vi "Dictionary Example.vi"() -> ()   [LabVIEW 2020]
uses:
  <userlib>/_OpenG.lib/dictionary/dictionary.llb/Dictionary Update (by scalar value)__ogtk.vi
  <userlib>/_OpenG.lib/string/string.llb/Trim Whitespace (String)__ogtk.vi
panel:
  in  "Copyright":bool
  in  "Help":bool
  in  "Cancel":bool
  in  "Delete Selected User":bool
  in  "Add":bool
  in  "New Username":string
  in  "Add New User":bool
  in  "Revert":bool
  in  "Exit":bool
  in  "Apply":bool
  in  "User Information":cluster{"Country":string, "Age":i32}
  out "error out":errorcluster
  in  "Selected User":u16(ring) items=["<Select Username>", "Tom", "Harish", "Sam", "Ghulam", "Henry", "Jon"]
  in  "error in (no error)":errorcluster
  # "Instructions to use the example:\n\n1. <Display User Information>\n     Select the User from \"Select User\" dropdown listbox\n     The information of that user will be displayed in \"User Information\" section\n\n2. <Modify User Information>\n     Select the User from \"Select User\" dropdown listbox\n     Modify the User Information\n     Click \"Apply Changes\" button to save\n\n3. <Revert User Information Changes>\n     Click \"Revert\" button to cancel the modifications\n\n3. <Add New User>\n    Click \"Add new user\" button\n    Enter the new user name in \"New Username\" button \n    Press \"+\" button to add       \n    the username to the dictionary\n\n4. <Delete Existing Username>\n     Select the username in \"Selected User\" listbox\n     Click \"Delete Selected User\" button\n     Select \"Yes\" in the confirmation dialog window\n\n5. <Exit>\n     Click \"Exit\" button to exit the application\n\n6. <Help>\n     Click \"Help\"button to see this help text in a dialog box."
  # "<Dictionary Example.vi> - <Demonstrates use of OpenG Dictionary functions>\n\nCopyright (C) 2005 Ashish Uttarwar <ashish.uttarwar@jameskring.com>\nCopyright (C) 2010 Jonathon Green <jg@jgcode.net>\n\nPlease visit http://www.OpenG.org to learn about the\nOpen Source LabVIEW software movement.\n\nThis library is free software; you can redistribute it and/or\nmodify it under the terms of the GNU Lesser General Public\nLicense as published by the Free Software Foundation; either\nversion 2.1 of the License, or (at your option) any later version.\nThis library is distributed in the hope that it will be useful,\nbut WITHOUT ANY WARRANTY; without even the implied warranty of\nMERCHANTABILITY or FITNESS FOR A PARTICULAR PURPOSE. See the GNU\nLesser General Public License for more details.\nYou should have received a copy of the GNU Lesser General Public\nLicense along with this library; if not, write to the Free Software\nFoundation, Inc., 59 Temple Place, Suite 330, Boston, MA 02111-1307 USA"
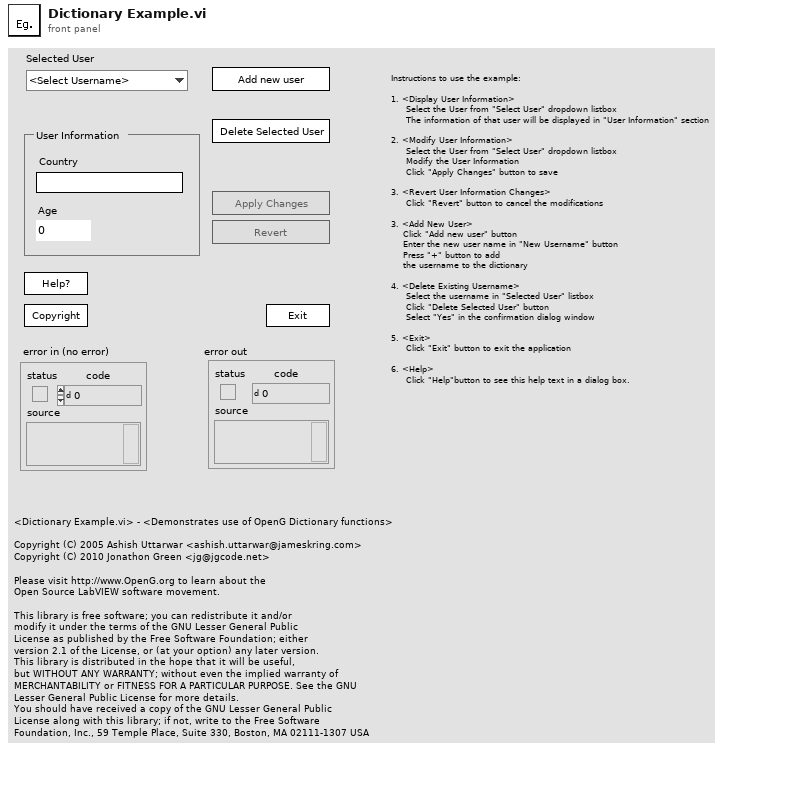
[diagram p1: front panel]
types:
  T1 = typedef "Dictionary Object RefNum__ogtk.ctl" = refnum<k1>
  T2 = cluster{"dictionary out":T1, "Selected Username":string, "Selected User Info":cluster{"Country":string, "Age":i32}, "Add/Delete Username":string}
  T3 = cluster{"Selected Username":string, "Value":cluster{"Country":string, "Age":i32}}
  T4 = cluster{"Username":string, "User_Info":cluster{"Country":string, "Age":i32}}[]
  T5 = cluster{"Add/Delete Username":string, "User Info Constant":cluster{"Country":string, "Age":i32}}
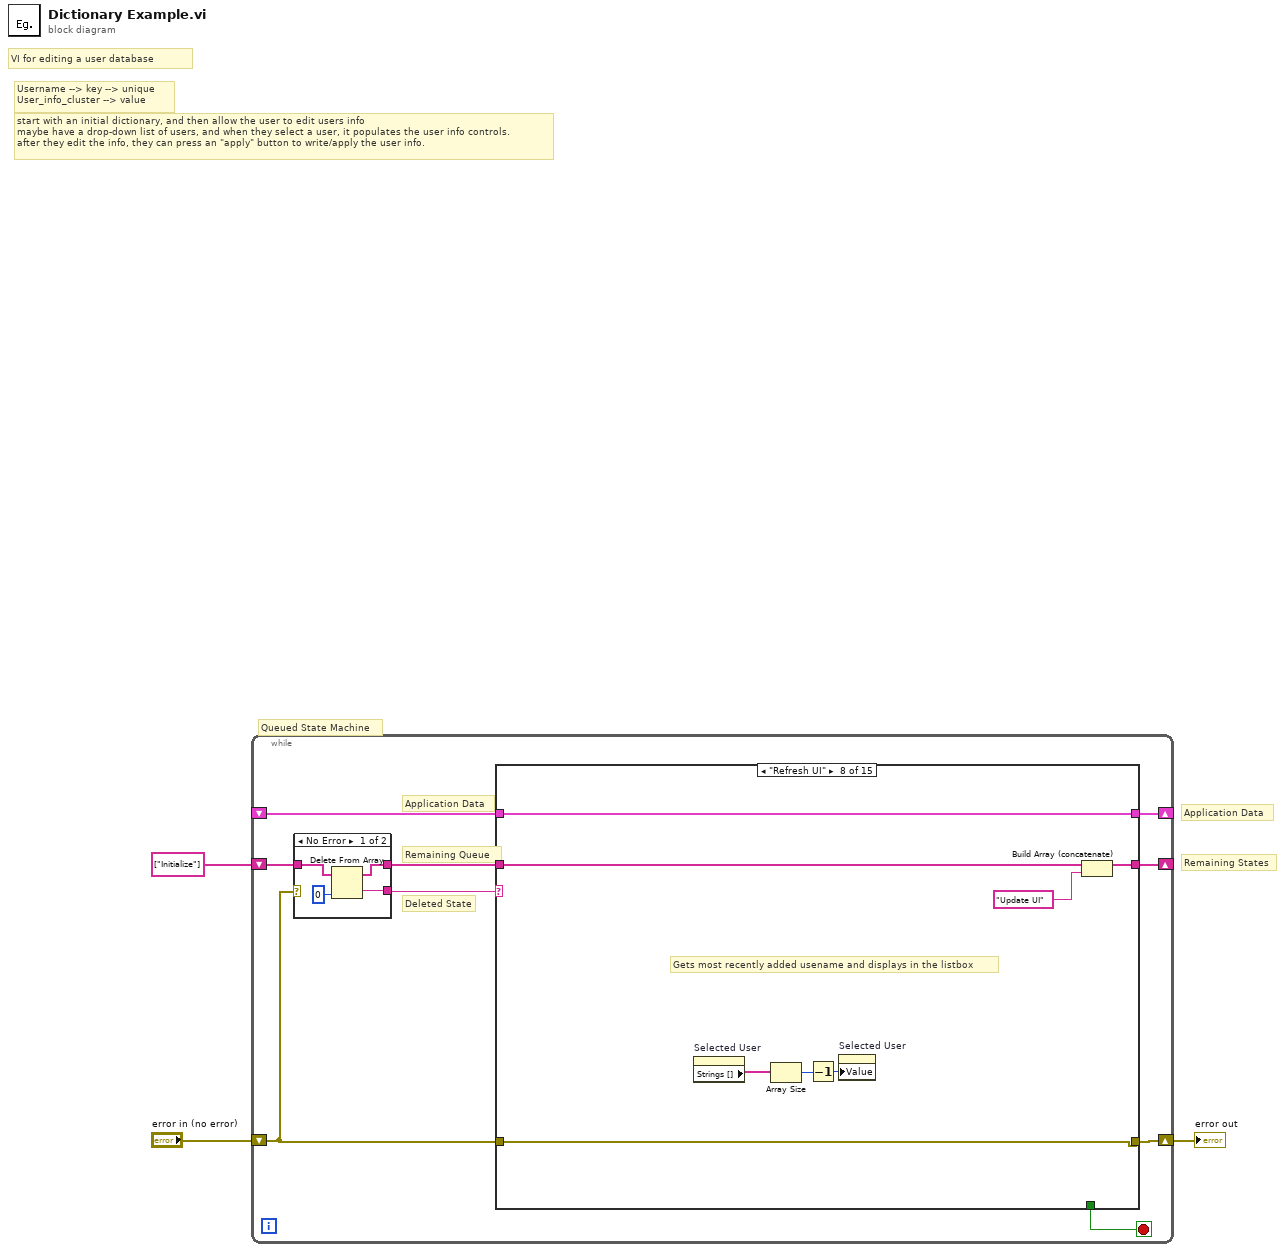
[diagram p0: block diagram]
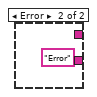
[diagram p2: hidden frame]
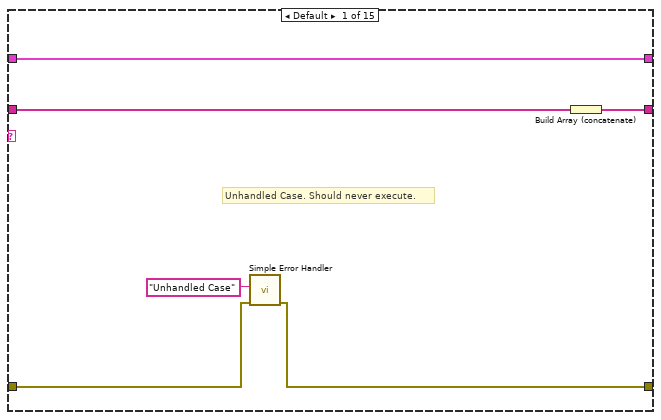
[diagram p3: hidden frame]
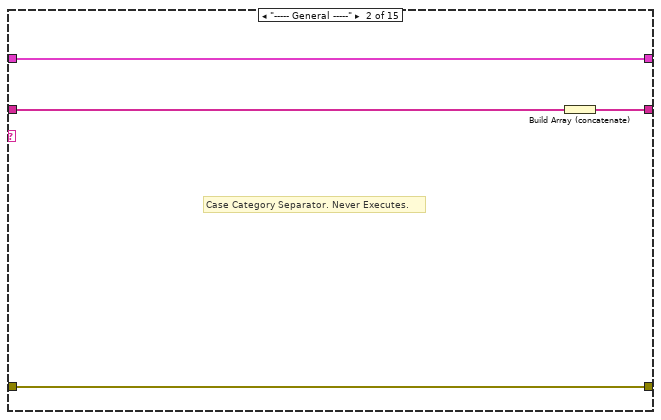
[diagram p4: hidden frame]
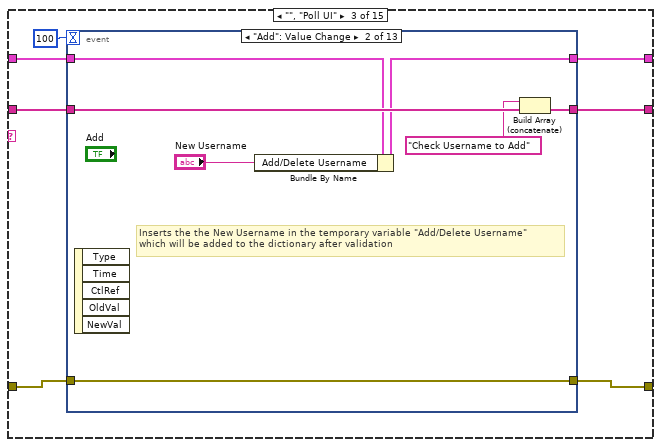
[diagram p5: hidden frame]
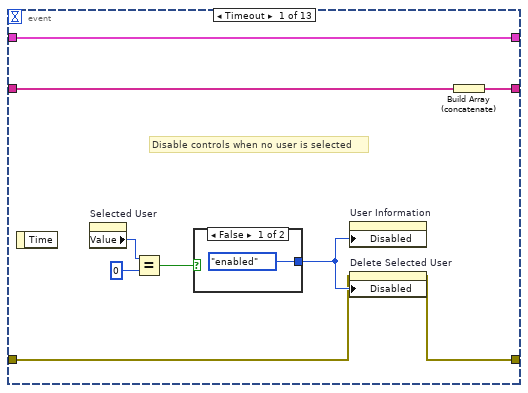
[diagram p6: hidden frame]
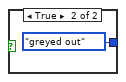
[diagram p7: hidden frame]
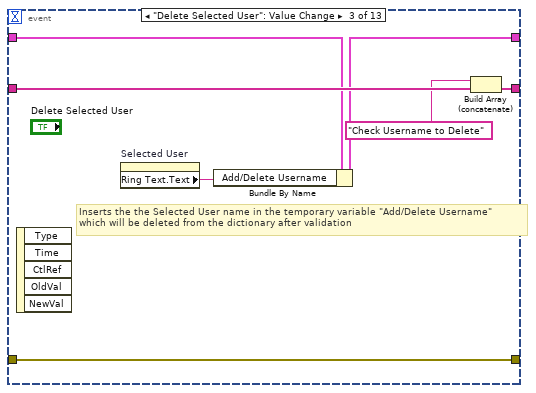
[diagram p8: hidden frame]
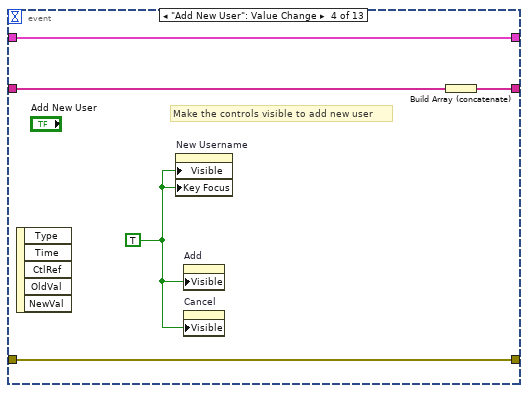
[diagram p9: hidden frame]
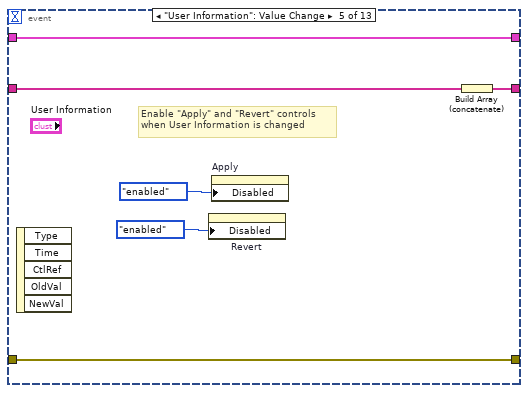
[diagram p10: hidden frame]
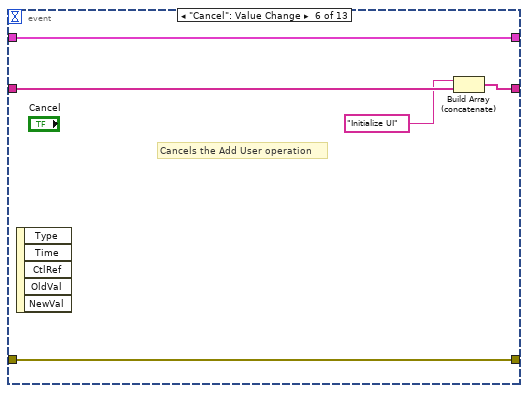
[diagram p11: hidden frame]
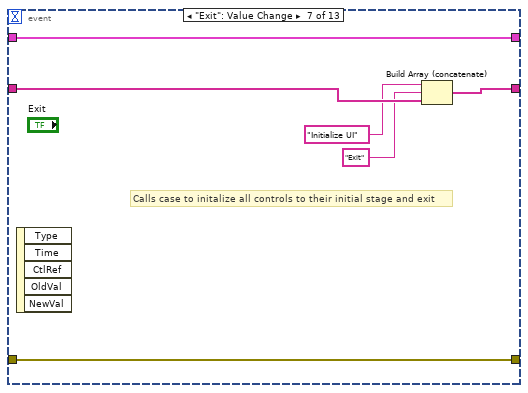
[diagram p12: hidden frame]
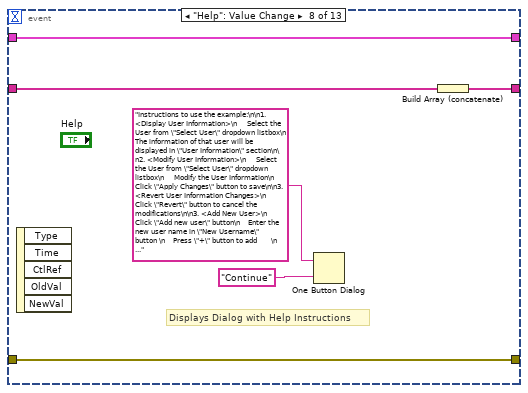
[diagram p13: hidden frame]
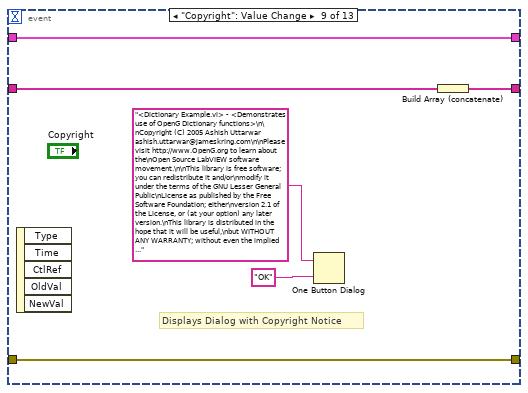
[diagram p14: hidden frame]
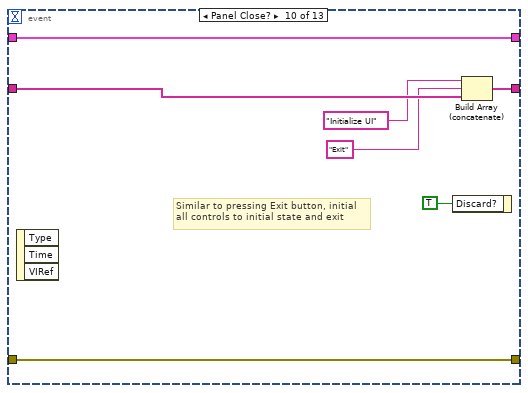
[diagram p15: hidden frame]
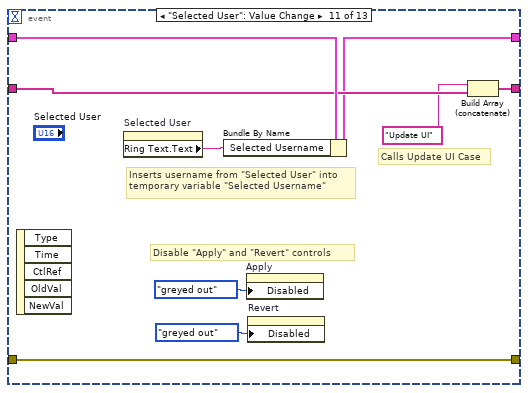
[diagram p16: hidden frame]
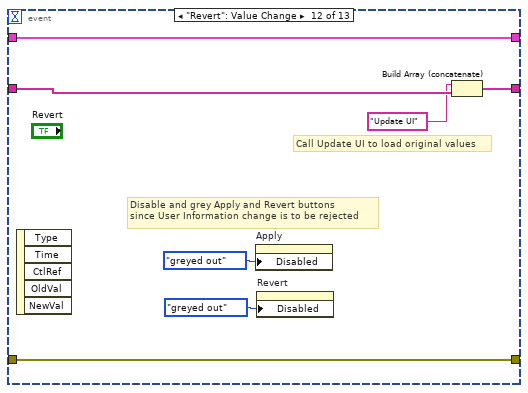
[diagram p17: hidden frame]
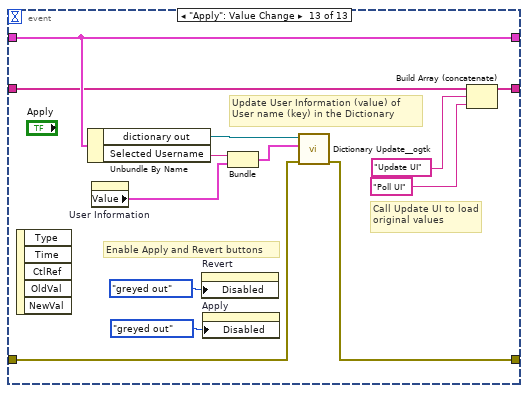
[diagram p18: hidden frame]
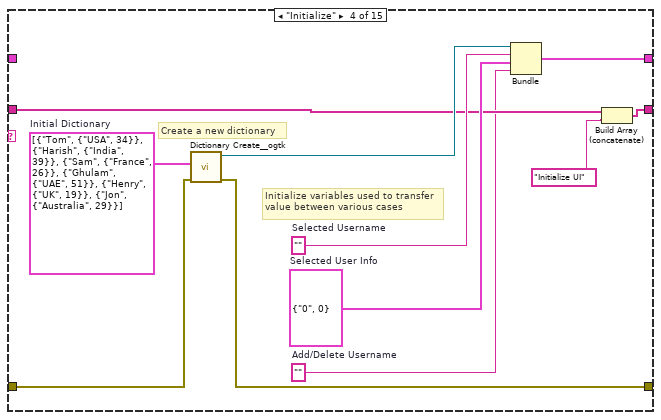
[diagram p19: hidden frame]
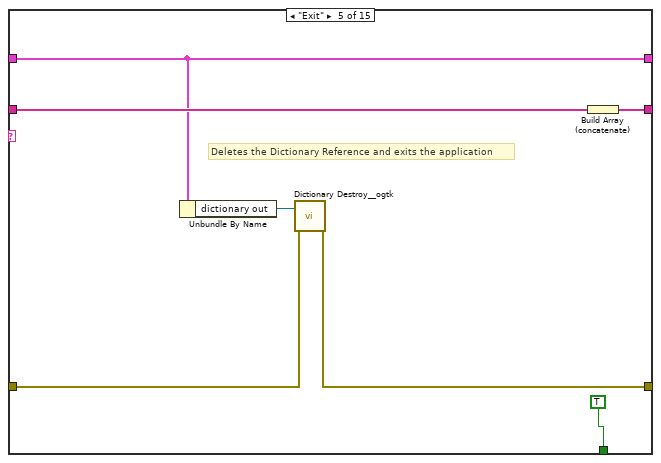
[diagram p20: hidden frame]
diagram:
  # "Queued State Machine"
  # "Remaining States"
  # "Application Data"
  # "Username --> key --> unique\nUser_info_cluster --> value"
  # "VI for editing a user database"
  # "start with an initial dictionary, and then allow the user to edit users info\nmaybe have a drop-down list of users, and when they select a user, it populates the user info controls.\nafter they edit the info, they can press an \"apply\" button to write/apply the user info."
  n1 = while {
    shift-right: [w12] -> _
    shift-left: _ -> [w9]
    shift-right: [w7] -> _
    shift-left: string[] ["Initialize"] -> [w11]
    shift-right: [w5] -> w2
    shift-left: "error in (no error)" -> [w4]
    stop <- w6 stop-if-true
    # "Deleted State"
    # "Remaining Queue"
    # "Application Data"
    n2 = case shown="No Error" w4 {
      tunnel: w11 -> [w16 _]
      tunnel: [w14 "Error" ("Ring Text.Text")] -> w10
      tunnel: [w13 _] -> w8
      frame No Error {
        n3 = Delete From Array(array=w16, index=0) -> (deleted portion=w14:string, array with subset deleted=w13:string[])  [unwired: 1 in]
      }
      frame Error {
      }
    }
    n4 = case shown="\"Refresh UI\"" w10 {
      tunnel: [w22 w26 w33 w138 w145 w150 w152 w178 w191 w201 w204 w238 w246 w250 w267] -> w12
      tunnel: w9 -> [w22 w26 w34 _ w145 w150 w152 w178 w191 w201 w204 w239 w246 w250 w266]
      tunnel: [w23 w27 w29 w140 w147 w151 w170 w181 w192 w202 w217 w243 w247 w257 w276] -> w7
      tunnel: w4 -> [w20 w24 w31 w134 w143 w148 w162 w177 w187 w199 w215 w231 w244 w255 w274]
      tunnel: [w19 w24 w32 w133 w142 w148 w158 w177 w184 w199 w206 w237 w244 w252 w273] -> w5
      tunnel: w8 -> [w21 w25 w30 w132 w146 w149 w161 w179 w182 w200 w216 w242 w245 w256 w275]
      tunnel: [_ _ _ _ TRUE _ _ _ _ _ _ _ _ _ _] -> w6
      frame Default {
        # "Unhandled Case. Should never execute."
        n5 = call <vilib>:"Simple Error Handler.vi"("error source (\" \")"="Unhandled Case" ("error source (\" \")"), "error in (no error)"=w20) -> ("error out"=w19:errorcluster)  [unwired: 3 in, 4 out]
        n6 = Build Array (concatenate)(w21) -> (w23:string[])
      }
      frame "----- General -----" {
        # "Case Category Separator. Never Executes."
        n7 = Build Array (concatenate)(w25) -> (w27:string[])
      }
      frame "", "Poll UI" {
        n8 = event shown="[1] \"Add\": Value Change" {
          selector: _ -> [_ _ _ _ _ _ _ _ _ _ _ _ _]
          dyn-events: _ -> [_ _ _ _ _ _ _ _ _ _ _ _ _]
          timeout: 100 -> [_ _ _ _ _ _ _ _ _ _ _ _ _]
          tunnel: w34 -> [w41 w47 w54 w64 w70 w75 w81 w87 w93 w100 w109 w110 w123]
          tunnel: [w41 w48 w55 w64 w70 w75 w81 w87 w93 w100 w101 w110 w123] -> w33
          tunnel: [w43 w52 w59 w63 w69 w74 w80 w86 w92 w99 w106 w115 w122] -> w29
          tunnel: w30 -> [w42 w50 w57 w61 w67 w72 w78 w84 w90 w97 w107 w116 w120]
          tunnel: [w37 w51 w58 w62 w68 w73 w79 w85 w91 w98 w104 w113 w124] -> w32
          tunnel: w31 -> [w35 w51 w58 w62 w68 w73 w79 w85 w91 w98 w104 w113 w125]
          event Timeout {
            # "Disable controls when no user is selected"
            n9 = event-data() -> ()  [unwired: 1 in, 1 out]
            n10 = property on="Selected User" class="Ring (strict)"() -> ("Value"=w40:u16)  [unwired: 2 in, 2 out]
            n11 = Equal?(x=w40, y=u16 0) -> (x = y?=w38:bool)
            n12 = case shown="False" w38 {
              tunnel: [enum16{"enabled", "disabled", "greyed out"}."enabled" enum16{"enabled", "disabled", "greyed out"}."greyed out"] -> w36
              frame False {
              }
              frame True {
              }
            }
            n13 = property on="User Information" class="Clust (strict)"("Disabled"=w36) -> ()  [unwired: 2 in, 2 out]
            n14 = property on="Delete Selected User" class="Bool"(error in=w35, "Disabled"=w36) -> (error out=w37:errorcluster)  [unwired: 1 in, 1 out]
            n15 = Build Array (concatenate)(w42) -> (w43:string[])
          }
          event "Add": Value Change {
            # "Inserts the the New Username in the temporary variable \"Add/Delete Username\" \nwhich will be added to the dictionary after validation"
            n16 = event-data() -> ()  [unwired: 1 in, 5 out]
            n17 = Bundle By Name(cluster=w47, "Add/Delete Username"="New Username") -> (w48:T2)
            n18 = Build Array (concatenate)("Check Username to Add" ("Ring Text.Text"), w50) -> (w52:string[])
          }
          event "Delete Selected User": Value Change {
            # "Inserts the the Selected User name in the temporary variable \"Add/Delete Username\" \nwhich will be deleted from the dictionary after validation"
            n19 = event-data() -> ()  [unwired: 1 in, 5 out]
            n20 = property on="Selected User" class="Ring (strict)"() -> ("Ring Text.Text"=w53:string)  [unwired: 2 in, 2 out]
            n21 = Bundle By Name(cluster=w54, "Add/Delete Username"=w53) -> (w55:T2)
            n22 = Build Array (concatenate)("Check Username to Delete" ("Ring Text.Text"), w57) -> (w59:string[])
          }
          event "Add New User": Value Change {
            w60 = TRUE ("Visible")
            # "Make the controls visible to add new user"
            n23 = event-data() -> ()  [unwired: 1 in, 5 out]
            n24 = property on="New Username" class="Str"("Visible"=w60, "Key Focus"=w60) -> ()  [unwired: 2 in, 2 out]
            n25 = property on="Add" class="Bool"("Visible"=w60) -> ()  [unwired: 2 in, 2 out]
            n26 = property on="Cancel" class="Bool"("Visible"=w60) -> ()  [unwired: 2 in, 2 out]
            n27 = Build Array (concatenate)(w61) -> (w63:string[])
          }
          event "User Information": Value Change {
            # "Enable \"Apply\" and \"Revert\" controls\nwhen User Information is changed"
            n28 = event-data() -> ()  [unwired: 1 in, 5 out]
            n29 = property on="Revert" class="Bool"("Disabled"=enum16{"enabled", "disabled", "greyed out"}."enabled") -> ()  [unwired: 2 in, 2 out]
            n30 = property on="Apply" class="Bool"("Disabled"=enum16{"enabled", "disabled", "greyed out"}."enabled") -> ()  [unwired: 2 in, 2 out]
            n31 = Build Array (concatenate)(w67) -> (w69:string[])
          }
          event "Cancel": Value Change {
            # "Cancels the Add User operation"
            n32 = event-data() -> ()  [unwired: 1 in, 5 out]
            n33 = Build Array (concatenate)("Initialize UI" ("Ring Text.Text"), w72) -> (w74:string[])
          }
          event "Exit": Value Change {
            # "Calls case to initalize all controls to their initial stage and exit"
            n34 = event-data() -> ()  [unwired: 1 in, 5 out]
            n35 = Build Array (concatenate)("Initialize UI" ("Ring Text.Text"), "Exit" ("Ring Text.Text"), w78) -> (w80:string[])
          }
          event "Help": Value Change {
            # "Displays Dialog with Help Instructions"
            n36 = event-data() -> ()  [unwired: 1 in, 5 out]
            n37 = One Button Dialog(message="Instructions to use the example:\n\n1. <Display User Information>\n     Select the User from \"Select User\" dropdown listbox\n     The information of that user will be displayed in \"User Information\" section\n\n2. <Modify User Information>\n     Select the User from \"Select User\" dropdown listbox\n     Modify the User Information\n     Click \"Apply Changes\" button to save\n\n3. <Revert User Information Changes>\n     Click \"Revert\" button to cancel the modifications\n\n3. <Add New User>\n    Click \"Add new user\" button\n    Enter the new user name in \"New Username\" button \n    Press \"+\" button to add       \n    the username to the dictionary\n\n4. <Delete Existing Username>\n     Select the username in \"Selected User\" listbox\n     Click \"Delete Selected User\" button\n     Select \"Yes\" in the confirmation dialog window\n\n5. <Exit>\n     Click \"Exit\" button to exit the application\n\n6. <Help>\n     Click \"Help\"button to see this help text in a dialog box.\n", button name ("OK")="Continue") -> ()  [unwired: 1 out]
            n38 = Build Array (concatenate)(w84) -> (w86:string[])
          }
          event "Copyright": Value Change {
            # "Displays Dialog with Copyright Notice"
            n39 = event-data() -> ()  [unwired: 1 in, 5 out]
            n40 = One Button Dialog(message="<Dictionary Example.vi> - <Demonstrates use of OpenG Dictionary functions>\n\nCopyright (C) 2005 Ashish Uttarwar ashish.uttarwar@jameskring.com\n\nPlease visit http://www.OpenG.org to learn about the\nOpen Source LabVIEW software movement.\n\nThis library is free software; you can redistribute it and/or\nmodify it under the terms of the GNU Lesser General Public\nLicense as published by the Free Software Foundation; either\nversion 2.1 of the License, or (at your option) any later version.\nThis library is distributed in the hope that it will be useful,\nbut WITHOUT ANY WARRANTY; without even the implied warranty of\nMERCHANTABILITY or FITNESS FOR A PARTICULAR PURPOSE. See the GNU\nLesser General Public License for more details.\nYou should have received a copy of the GNU Lesser General Public\nLicense along with this library; if not, write to the Free Software\nFoundation, Inc., 59 Temple Place, Suite 330, Boston, MA 02111-1307 USA", button name ("OK")="OK") -> ()  [unwired: 1 out]
            n41 = Build Array (concatenate)(w90) -> (w92:string[])
          }
          event Panel Close? {
            # "Similar to pressing Exit button, initial\nall controls to initial state and exit"
            n42 = event-data() -> ()  [unwired: 1 in, 3 out]
            n43 = event-data("Discard?"=TRUE) -> ()  [unwired: 1 in, 1 out]
            n44 = Build Array (concatenate)("Initialize UI" ("Ring Text.Text"), "Exit" ("Ring Text.Text"), w97) -> (w99:string[])
          }
          event "Selected User": Value Change {
            # "Calls Update UI Case"
            # "Disable \"Apply\" and \"Revert\" controls"
            # "Inserts username from \"Selected User\" into\ntemporary variable \"Selected Username\""
            n45 = event-data() -> ()  [unwired: 1 in, 5 out]
            n46 = property on="Selected User" class="Ring (strict)"() -> ("Ring Text.Text"=w108:string)  [unwired: 2 in, 2 out]
            n47 = Bundle By Name(cluster=w109, "Selected Username"=w108) -> (w101:T2)
            n48 = property on="Apply" class="Bool"("Disabled"=enum16{"enabled", "disabled", "greyed out"}."greyed out") -> ()  [unwired: 2 in, 2 out]
            n49 = property on="Revert" class="Bool"("Disabled"=enum16{"enabled", "disabled", "greyed out"}."greyed out") -> ()  [unwired: 2 in, 2 out]
            n50 = Build Array (concatenate)("Update UI" ("element"), w107) -> (w106:string[])
          }
          event "Revert": Value Change {
            # "Call Update UI to load original values"
            # "Disable and grey Apply and Revert buttons\nsince User Information change is to be rejected"
            n51 = event-data() -> ()  [unwired: 1 in, 5 out]
            n52 = property on="Apply" class="Bool"("Disabled"=enum16{"enabled", "disabled", "greyed out"}."greyed out") -> ()  [unwired: 2 in, 2 out]
            n53 = property on="Revert" class="Bool"("Disabled"=enum16{"enabled", "disabled", "greyed out"}."greyed out") -> ()  [unwired: 2 in, 2 out]
            n54 = Build Array (concatenate)("Update UI" ("element"), w116) -> (w115:string[])
          }
          event "Apply": Value Change {
            # "Update User Information (value) of  \nUser name (key) in the Dictionary"
            # "Enable Apply and Revert buttons"
            # "Call Update UI to load original values"
            n55 = event-data() -> ()  [unwired: 1 in, 5 out]
            n56 = Unbundle By Name(w123) -> ("dictionary out"=w129:T1, "Selected Username"=w128:string)
            n57 = property on="User Information" class="Clust (strict)"() -> ("Value"=w127:cluster{"Country":string, "Age":i32})  [unwired: 2 in, 2 out]
            n58 = property on="Revert" class="Bool"("Disabled"=enum16{"enabled", "disabled", "greyed out"}."greyed out") -> ()  [unwired: 2 in, 2 out]
            n59 = property on="Apply" class="Bool"("Disabled"=enum16{"enabled", "disabled", "greyed out"}."greyed out") -> ()  [unwired: 2 in, 2 out]
            n60 = Bundle("Selected Username"=w128, "Value"=w127) -> (w126:T3)  [unwired: 1 in]
            n61 = call-poly <userlib>:"Dictionary Update__ogtk.vi"("error in (no error)"=w125, "key-value"=w126, "dictionary"=w129) -> ("error out"=w124:errorcluster)  [unwired: 6 in, 2 out]
            n62 = Build Array (concatenate)(w120, "Update UI" ("Ring Text.Text"), "Poll UI" ("Ring Text.Text")) -> (w122:string[])
          }
        }
      }
      frame "Initialize" {
        w130 = T4 [{"Username"="Tom", "User_Info"={"Country"="USA", "Age"=34}}, {"Username"="Harish", "User_Info"={"Country"="India", "Age"=39}}, {"Username"="Sam", "User_Info"={"Country"="France", "Age"=26}}, {"Username"="Ghulam", "User_Info"={"Country"="UAE", "Age"=51}}, {"Username"="Henry", "User_Info"={"Country"="UK", "Age"=19}}, {"Username"="Jon", "User_Info"={"Country"="Australia", "Age"=29}}]  # Initial Dictionary
        w137 = cluster{"Country":string, "Age":i32} {"Country"="0", "Age"=0}  # Selected User Info
        w131 = ""  # Add/Delete Username
        w139 = ""  # Selected Username
        # "Initialize variables used to transfer\nvalue between various cases"
        # "Create a new dictionary"
        n63 = call <userlib>:"Dictionary Create__ogtk.vi"("error in (no error)"=w134, "initial dictionary (empty)"=w130) -> ("error out"=w133:errorcluster, "dictionary out"=w135:T1)  [unwired: 8 in]
        n64 = Bundle("dictionary out"=w135, "Selected Username"=w139, "Selected User Info"=w137, "Add/Delete Username"=w131) -> (w138:T2)  [unwired: 1 in]
        n65 = Build Array (concatenate)(w132, "Initialize UI" ("Ring Text.Text")) -> (w140:string[])
      }
      frame "Exit" {
        # "Deletes the Dictionary Reference and exits the application"
        n66 = Unbundle By Name(w145) -> ("dictionary out"=w144:T1)
        n67 = call <userlib>:"Dictionary Destroy__ogtk.vi"("error in (no error)"=w143, "dictionary"=w144) -> ("error out"=w142:errorcluster)  [unwired: 9 in]
        n68 = Build Array (concatenate)(w146) -> (w147:string[])
      }
      frame "----- UI -----" {
        # "Case Category Separator. Never Executes."
        n69 = Build Array (concatenate)(w149) -> (w151:string[])
      }
      frame "Initialize UI" {
        w160 = u16 0 items=["<Select Username>", "Tom", "Harish", "Sam", "Ghulam", "Henry"] ("Selected Username")
        w153 = FALSE ("Visible")
        # "Gets all Usernames (keys) from the\ndictionary and populate tme in the listbox"
        # "Initialize controls and indicators with default values"
        n70 = Unbundle By Name(w152) -> ("dictionary out"=w163:T1)
        n71 = property on="New Username" class="Str"("Visible"=w153) -> ()  [unwired: 2 in, 2 out]
        n72 = property on="New Username" class="Str"("Text.Text"="") -> ()  [unwired: 2 in, 2 out]
        n73 = property on="Add" class="Bool"("Visible"=w153) -> ()  [unwired: 2 in, 2 out]
        n74 = property on="Cancel" class="Bool"("Visible"=w153) -> ()  [unwired: 2 in, 2 out]
        n75 = call <userlib>:"Dictionary Get Keys__ogtk.vi"("error in (no error)"=w162, "dictionary"=w163) -> ("error out"=w169:errorcluster, "keys"=w168:variant[])  [unwired: 7 in, 1 out]
        n76 = for {
          tunnel: w168 -> [w173] mode=indexing
          tunnel: [w171] -> w167 mode=indexing
          n77 = Variant To Data(type="" ("String"), Variant=w173) -> (data=w171:string)  [unwired: 1 in, 1 out]
        }
        n78 = property on="Revert" class="Bool"("Disabled"=enum16{"enabled", "disabled", "greyed out"}."greyed out") -> ()  [unwired: 2 in, 2 out]
        n79 = property on="Apply" class="Bool"("Disabled"=enum16{"enabled", "disabled", "greyed out"}."greyed out") -> ()  [unwired: 2 in, 2 out]
        n80 = property on="User Information" class="Clust (strict)"("Value"=cluster{"Country":string, i32} {"Country"="", 0} ("User Information")) -> ()  [unwired: 2 in, 2 out]
        n81 = Build Array (concatenate)("<Select Username>" ("Ring Text.Text"), w167) -> (w166:string[])
        n82 = property on="Selected User" class="Ring (strict)"(error in=w169, "Strings []"=w166) -> (error out=w159:errorcluster)  [unwired: 1 in, 1 out]
        n83 = property on="Selected User" class="Ring (strict)"(error in=w159, "Value"=w160) -> (error out=w158:errorcluster)  [unwired: 1 in, 1 out]
        n84 = Build Array (concatenate)(w161, "Update UI" ("Ring Text.Text")) -> (w170:string[])
      }
      frame "Refresh UI" {
        # "Gets most recently added usename and displays in the listbox"
        n85 = property on="Selected User" class="Ring (strict)"() -> ("Strings []"=w176:string[])  [unwired: 2 in, 2 out]
        n86 = Array Size(array=w176) -> (size(s)=w175:i32)
        n87 = Decrement(x=w175) -> (x-1=w174:i32)
        n88 = property on="Selected User" class="Ring (strict)"("Value"=w174) -> ()  [unwired: 2 in, 2 out]
        n89 = Build Array (concatenate)(w179, "Update UI" ("Ring Text.Text")) -> (w181:string[])
      }
      frame "Update UI" {
        # "Check if Selected Usename is\npresent in dictionary"
        n90 = Unbundle By Name(w191) -> ("dictionary out"=w188:T1, "Selected Username"=w189:string)
        n91 = call <userlib>:"Dictionary Get Value__ogtk.vi"("error in"=w187, "key"=w189, "dictionary"=w188) -> ("error out"=w185:errorcluster, "found?"=w183:bool, "value"=w186:variant)  [unwired: 5 in, 1 out]
        n92 = case shown="True" w183 {
          tunnel: w186 -> [_ w197]
          tunnel: w185 -> [w193 w195]
          tunnel: [w193 w194] -> w184
          frame False {
          }
          frame True {
            w198 = cluster{"Country":string, "Age":i32} {"Country"="", "Age"=0}  # User_Info
            n93 = Variant To Data(error in=w195, type=w198, Variant=w197) -> (data=w196:cluster{"Country":string, "Age":i32}, error out=w194:errorcluster)
            n94 = property on="User Information" class="Clust (strict)"("Value"=w196) -> ()  [unwired: 2 in, 2 out]
          }
        }
        n95 = Build Array (concatenate)(w182, "Poll UI" ("Ring Text.Text")) -> (w192:string[])
      }
      frame "----- Add -----" {
        # "Case Category Separator. Never Executes."
        n96 = Build Array (concatenate)(w200) -> (w202:string[])
      }
      frame "Check Username to Add" {
        # "Username\nNot Empty?"
        # "Username\nNot Present?"
        n97 = Unbundle By Name(w204) -> ("Add/Delete Username"=w203:string, "dictionary out"=w214:T1)
        n98 = call <userlib>:"Dictionary Get Value__ogtk.vi"("error in"=w215, "key"=w203, "dictionary"=w214) -> ("error out"=w205:errorcluster, "found?"=w209:bool)  [unwired: 5 in, 2 out]
        n99 = call-poly <userlib>:"Trim Whitespace__ogtk.vi"("Remove (leading and trailing)"=enum16{"leading", "trailing", "both"}."both" ("remove (leading and trailing)"), "String in"=w203) -> ("String out"=w212:string)  [unwired: 5 in]
        n100 = Not(x=w209) -> (.not. x?=w208:bool)
        n101 = Not Equal?(x=w212, y="") -> (x != y?=w210:bool)
        n102 = case shown="True" w210 {
          tunnel: w208 -> [_ w224]
          tunnel: ["Initialize UI" ("Ring Text.Text") w223] -> w207
          tunnel: [w218 w222] -> w206
          tunnel: w205 -> [w218 w221]
          frame False {
            # "New Username supplied is NOT VALID (empty)."
            n103 = One Button Dialog(message="Invalid username (empty value)") -> ()  [unwired: 1 in, 1 out]
          }
          frame True {
            n104 = case shown="True" w224 {
              tunnel: ["Initialize UI" ("Ring Text.Text") "Add Username" ("Ring Text.Text")] -> w223
              tunnel: [w225 w228] -> w222
              tunnel: w221 -> [w225 w228]
              frame False {
                # "New Username supplied is NOT VALID (found in the dictionary)."
                n105 = One Button Dialog(message="Username \nalready exists.") -> ()  [unwired: 1 in, 1 out]
              }
              frame True {
                # "Username supplied is VALID (not empty and not found in the dictionary)."
              }
            }
          }
        }
        n106 = Build Array (concatenate)(w207, w216) -> (w217:string[])
      }
      frame "Add Username" {
        w241 = cluster{"Country":string, "Age":i32} {"Country"="", "Age"=0}  # User Info Constant
        # "Insert username and information in variables\nto pass to other cases being called"
        # "Update the Username (key) with\nempty User Information (values)"
        n107 = Unbundle By Name(w239) -> ("Add/Delete Username"=w234:string, "dictionary out"=w230:T1)
        n108 = Bundle("Add/Delete Username"=w234, "User Info Constant"=w241) -> (w240:T5)  [unwired: 1 in]
        n109 = Unbundle By Name(w240) -> ("Add/Delete Username"=w236:string, "User Info Constant"=w235:cluster{"Country":string, "Age":i32})
        n110 = call-poly <userlib>:"Dictionary Update__ogtk.vi"("error in (no error)"=w231, "key-value"=w240, "dictionary"=w230) -> ("error out"=w237:errorcluster)  [unwired: 6 in, 2 out]
        n111 = Bundle By Name(cluster=w239, "Selected Username"=w236, "Selected User Info"=w235) -> (w238:T2)
        n112 = Build Array (concatenate)("Initialize UI" ("Ring Text.Text"), "Refresh UI" ("Ring Text.Text"), w242) -> (w243:string[])
      }
      frame "----- Delete -----" {
        # "Case Category Separator. Never Executes."
        n113 = Build Array (concatenate)(w245) -> (w247:string[])
      }
      frame "Check Username to Delete" {
        # "Username\nPresent?"
        n114 = Unbundle By Name(w250) -> ("dictionary out"=w254:T1, "Add/Delete Username"=w248:string)
        n115 = call <userlib>:"Dictionary Get Value__ogtk.vi"("error in"=w255, "key"=w248, "dictionary"=w254) -> ("error out"=w251:errorcluster, "found?"=w249:bool)  [unwired: 5 in, 2 out]
        n116 = case shown="False" w249 {
          tunnel: ["Initialize UI" ("Ring Text.Text") "Delete User" ("Ring Text.Text")] -> w253
          tunnel: [w259 w261] -> w252
          tunnel: w251 -> [w259 w261]
          frame False {
            # "New Username supplied is NOT VALID (not found in the dictionary)."
            n117 = One Button Dialog(message="Usename is not valid." ("Ring Text.Text")) -> ()  [unwired: 1 in, 1 out]
          }
          frame True {
            # "Username supplied is present in the dictionary. Hence delete it."
          }
        }
        n118 = Build Array (concatenate)(w253, w256) -> (w257:string[])
      }
      frame "Delete User" {
        # "Confirm before deleting the \nuser from the dictionary"
        n119 = Unbundle By Name(w266) -> ("dictionary out"=w265:T1, "Add/Delete Username"=w264:string)
        n120 = Two Button Dialog(message="Are you sure?", 1:"No" ("F button name (\"Cancel\")"), 2:"Yes" ("T button name (\"OK\")")) -> (T button?=w271:bool)
        n121 = case shown="True" w271 {
          tunnel: w274 -> [w277 w281]
          tunnel: [w277 w280] -> w273
          tunnel: w265 -> [_ w279]
          tunnel: w264 -> [_ w278]
          frame False {
          }
          frame True {
            # "Delete the username (key) and user\ninformation (value) from dictionary"
            n122 = call <userlib>:"Dictionary Delete Element__ogtk.vi"("error in (no error)"=w281, "key"=w278, "dictionary"=w279) -> ("error out"=w280:errorcluster)  [unwired: 7 in, 1 out]
          }
        }
        n123 = Bundle By Name(cluster=w266, "Selected Username"="<Select Username>") -> (w267:T2)
        n124 = Build Array (concatenate)("Initialize UI" ("Ring Text.Text"), w275) -> (w276:string[])
      }
    }
  }
  "error out" <- w2
